vi "Initialize FLS Laser.vi"(4 "Fault?":bool, 6 "FLS Laser ID (A,B,C or D)":enum16{"A", "B", "C", "D"}(ring), 7 "FLS Status LEDs Refnum":refnum<vi>, 8 "error in (no error)":errorcluster, 9 "FLS Range Refnum":refnum<vi>, 10 "FLS COM Port":refnum<visa-resource-name>, 11 "FLS Laser Actor in":refnum<class "FLS Laser Actor.lvclass">) -> (0 "error out":errorcluster, 3 "DLS Laser Actor out":refnum<class "FLS Laser Actor.lvclass">)   [LabVIEW 2018, in "FLS Laser Actor.lvlib" / "FLS Laser Actor.lvclass"]
uses:
  FLS Laser Actor.lvclass
  C:/Program Files (x86)/National Instruments/LabVIEW 2018/vi.lib/ActorFramework/Actor/Actor.lvclass
  FLS Laser Actor.lvclass/FLS Laser Actor.ctl
  <vilib>/ActorFramework/Actor/Actor.lvclass/Actor.ctl
  <vilib>/ActorFramework/Message Enqueuer/Message Enqueuer.lvclass/Message Enqueuer.ctl
  <vilib>/ActorFramework/Message Enqueuer/Init from Existing Queue.vi
  <vilib>/ActorFramework/Message Enqueuer/Enqueue.vi
  <vilib>/ActorFramework/Stop Msg/Stop Msg.lvclass
  C:/Program Files (x86)/National Instruments/LabVIEW 2018/vi.lib/ActorFramework/Message/Message.lvclass
  <vilib>/Instr/_visa.llb/VISA Configure Serial Port (Instr).vi
  <vilib>/ActorFramework/Message Priority Queue/Priority Enqueue.vi
  <vilib>/ActorFramework/Message Enqueuer/Message Enqueuer.lvclass
  <vilib>/ActorFramework/Actor/Actor.lvclass
  Range Controller Actor Messages/Send Log Message to Caller Msg/Send Log Message to Caller Msg.lvclass
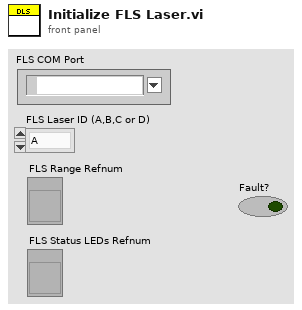
[diagram p1: front panel]
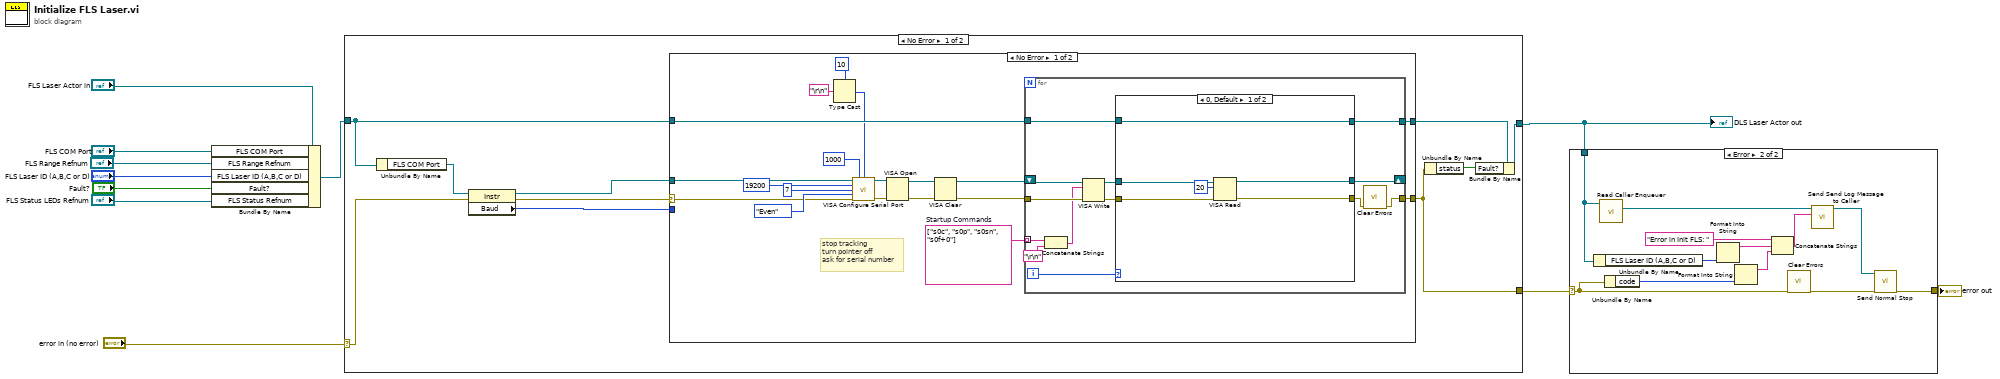
[diagram p0: block diagram]
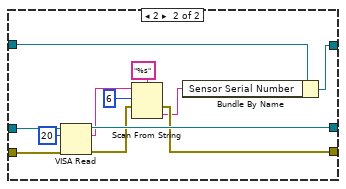
[diagram p3: hidden frame]
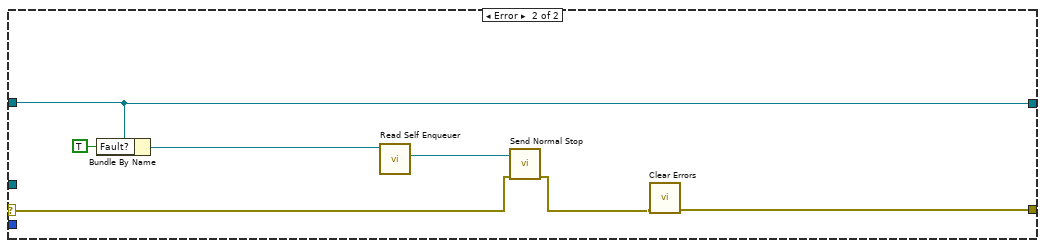
[diagram p4: hidden frame]
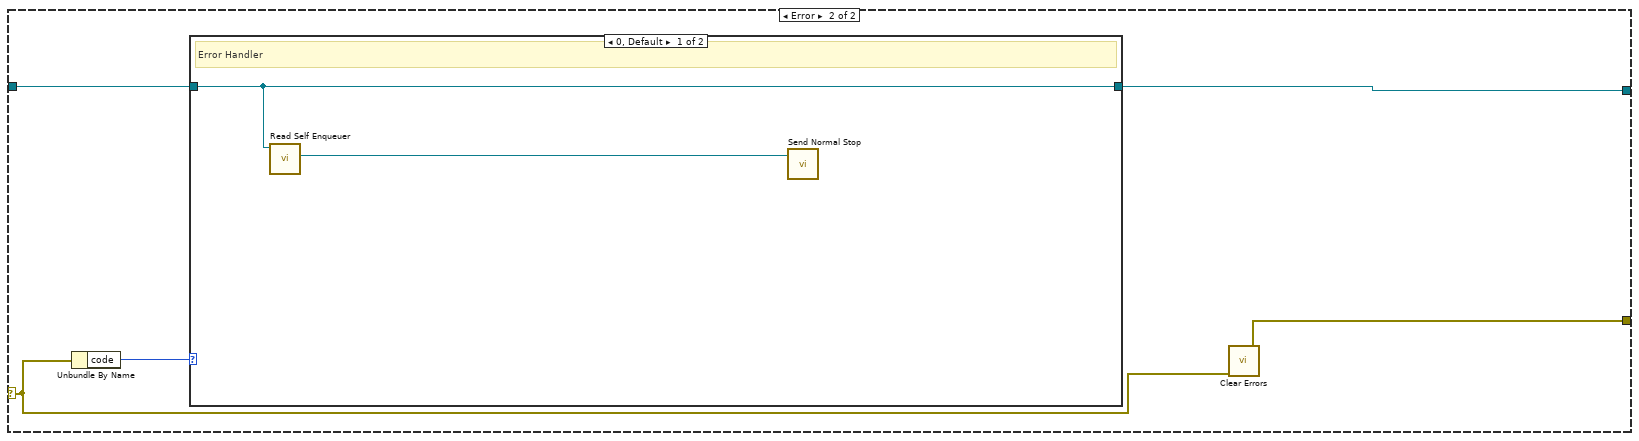
[diagram p5: hidden frame]
diagram:
  n1 = Bundle By Name(cluster="FLS Laser Actor in", "FLS COM Port"="FLS COM Port", "FLS Range Refnum"="FLS Range Refnum", "FLS Laser ID (A,B,C or D)"="FLS Laser ID (A,B,C or D)", "Fault?"="Fault?", "FLS Status Refnum"="FLS Status LEDs Refnum") -> (w10:refnum<class "FLS Laser Actor.lvclass">)
  n2 = case shown="No Error" "error in (no error)" {
    selector: "error in (no error)" -> [w17 w80]
    tunnel: [w13 w82] -> w2
    tunnel: [w15 w81] -> w3
    tunnel: w10 -> [w21 w83]
    frame No Error {
      n3 = Unbundle By Name(w21) -> ("FLS COM Port"=w20:refnum<visa-resource-name>)
      n4 = property class="Instr"(reference=w20, error in=w17) -> (reference out=w18:refnum<visa-resource-name>, error out=w19:errorcluster, "Baud"=w14:u32)
      n5 = case shown="No Error" w19 {
        selector: w19 -> [w26 w75]
        tunnel: [w40 w74] -> w16
        tunnel: w21 -> [w39 w74]
        tunnel: [w38 w77] -> w13
        tunnel: w18 -> [w23 _]
        tunnel: w14 -> [_ _]
        frame No Error {
          w27 = string[] ["s0c", "s0p", "s0sn", "s0f+0"]  # Startup Commands
          # "stop tracking\nturn pointer off\nask for serial number"
          n6 = Type Cast(type=u8 10 ("termination char\n(0xA = '\\n' = LF)"), x="\r\n") -> (*(type *) &x=w33:u8)
          n7 = call-poly "VISA Configure Serial Port"("VISA resource name"=w23, "timeout (10sec)"=u32 1000, "termination char\n(0xA = '\\n' = LF)"=w33, "baud rate (9600)"=u32 19200, "data bits (8)"=u16 7, "parity (0:none)"=enum16{"None", "Odd", "Even", "Mark", "Space"}."Even", "error in (no error)"=w26) -> ("VISA resource name out"=w24:refnum<visa-resource-name>, "error out"=w25:errorcluster)  [unwired: 7 in]
          n8 = VISA Open(error in (no error)=w25, VISA resource name=w24) -> (VISA resource name=w35:refnum<visa-resource-name>, error out=w37:errorcluster)  [unwired: 3 in]
          n9 = VISA Clear(VISA resource name=w35, error in (no error)=w37) -> (VISA resource name out=w34:refnum<visa-resource-name>, error out=w36:errorcluster)
          n10 = for {
            tunnel: w36 -> [w44]
            tunnel: w27 -> [w50] mode=indexing
            tunnel: w39 -> [w52]
            tunnel: [w51] -> w40
            tunnel: [w46] -> w38
            shift-right: [w48] -> _
            shift-left: w34 -> [w45]
            i -> [w53]
            n11 = Concatenate Strings(w50, "\r\n") -> (w41:string)
            n12 = VISA Write(VISA resource name=w45, write buffer=w41, error in (no error)=w44) -> (VISA resource name out=w43:refnum<visa-resource-name>, error out=w42:errorcluster)  [unwired: 1 out]
            n13 = case shown="0, Default" w53 {
              tunnel: w42 -> [w57 w70]
              tunnel: w43 -> [w58 w69]
              tunnel: w52 -> [w59 w67]
              tunnel: [w59 w66] -> w51
              tunnel: [w54 w63] -> w47
              tunnel: [w56 w71] -> w48
              frame 0, Default {
                n14 = VISA Read(VISA resource name=w58, byte count=u32 20, error in (no error)=w57) -> (VISA resource name out=w56:refnum<visa-resource-name>, error out=w54:errorcluster)  [unwired: 2 out]
              }
              frame 2 {
                n15 = VISA Read(VISA resource name=w69, byte count=u32 20, error in (no error)=w70) -> (VISA resource name out=w71:refnum<visa-resource-name>, read buffer=w62:string, error out=w64:errorcluster)  [unwired: 1 out]
                n16 = Scan From String(format string="%s", input string=w62, initial scan location=u32 6, error in=w64) -> (error out=w63:errorcluster, output 1=w60:string)  [unwired: 1 in, 2 out]
                n17 = Bundle By Name(cluster=w67, "Sensor Serial Number"=w60) -> (w66:refnum<class "FLS Laser Actor.lvclass">)
              }
            }
            n18 = call <vilib>:"Clear Errors.vi"("error in (no error)"=w47) -> ("error out"=w46:errorcluster)  [unwired: 5 in, 1 out]
          }
        }
        frame Error {
          n19 = Bundle By Name(cluster=w74, "Fault?"=TRUE) -> (w72:refnum<class "FLS Laser Actor.lvclass">)
          n20 = call <vilib>:"Read Self Enqueuer.vi"("Actor"=w72) -> ("Self Enqueuer"=w78:refnum<class "Message Enqueuer.lvclass">)  [unwired: 10 in]
          n21 = call <vilib>:"Send Normal Stop.vi"("error in (no error)"=w75, "Message Enqueuer"=w78) -> ("error out"=w76:errorcluster)  [unwired: 9 in]
          n22 = call <vilib>:"Clear Errors.vi"("error in (no error)"=w76) -> ("error out"=w77:errorcluster)  [unwired: 5 in, 1 out]
        }
      }
      n23 = Unbundle By Name(w13) -> ("status"=w12:bool)
      n24 = Bundle By Name(cluster=w16, "Fault?"=w12) -> (w15:refnum<class "FLS Laser Actor.lvclass">)
    }
    frame Error {
      n25 = Unbundle By Name(w80) -> ("code"=w79:i32)
      n26 = case shown="0, Default" w79 {
        tunnel: w83 -> [w84 w86]
        tunnel: [w84 w86] -> w81
        frame 0, Default {
          # "Error Handler"
          n27 = call <vilib>:"Read Self Enqueuer.vi"("Actor"=w84) -> ("Self Enqueuer"=w85:refnum<class "Message Enqueuer.lvclass">)  [unwired: 10 in]
          n28 = call <vilib>:"Send Normal Stop.vi"("Message Enqueuer"=w85) -> ()  [unwired: 10 in, 1 out]
        }
        frame 1 {
        }
      }
      n29 = call <vilib>:"Clear Errors.vi"("error in (no error)"=w80) -> ("error out"=w82:errorcluster)  [unwired: 5 in, 1 out]
    }
  }
  "DLS Laser Actor out" <- w3
  n30 = case shown="Error" w2 {
    selector: w2 -> [w87 w88]
    tunnel: w3 -> [_ w98]
    tunnel: [w87 w92] -> w1
    frame No Error {
    }
    frame Error {
      n31 = Unbundle By Name(w98) -> ("FLS Laser ID (A,B,C or D)"=w97:enum16{"A", "B", "C", "D"})
      n32 = call <vilib>:"Read Caller Enqueuer.vi"("Actor"=w98) -> ("Caller Enqueuer"=w99:refnum<class "Message Enqueuer.lvclass">)  [unwired: 10 in]
      n33 = Unbundle By Name(w88) -> ("code"=w90:i32)
      n34 = Format Into String(w97) -> (resulting string=w95:string)  [unwired: 3 in, 1 out]
      n35 = Format Into String(w90) -> (resulting string=w89:string)  [unwired: 3 in, 1 out]
      n36 = Concatenate Strings("Error in Init FLS: " ("Log Message"), w95, w89) -> (w91:string)
      n37 = call <vilib>:"Clear Errors.vi"("error in (no error)"=w88) -> ("error out"=w93:errorcluster)  [unwired: 5 in, 1 out]
      n38 = call "Send Send Log Message to Caller.vi"("Log Message"=w91, "Message Enqueuer in"=w99) -> ("Message Enqueuer out"=w94:refnum<class "Message Enqueuer.lvclass">)  [unwired: 8 in, 1 out]
      n39 = call <vilib>:"Send Normal Stop.vi"("error in (no error)"=w93, "Message Enqueuer"=w94) -> ("error out"=w92:errorcluster)  [unwired: 9 in]
    }
  }
  "error out" <- w1
